vi "Measurement Logic.vi"() -> ()   [LabVIEW 2024, in "NIScopeTimeDomain.lvlib"]
uses:
  NIScopeTimeDomain.lvlib
  Measurement Configuration.ctl
  <vilib>/MeasurementLink/MeasurementLink Measurement Server/Measure Call Context/Measure Call Context.lvclass
  Measurement Results.ctl
  <instrlib>/niScope/Controls/niScope scalar measurement.ctl
  <vilib>/MeasurementLink/MeasurementLink Measurement Server/Measure Call Context/Reserve Sessions - 1Pin.vi
  <vilib>/MeasurementLink/MeasurementLink niScope/Initialize Sessions - 1Sess.vi
  <vilib>/MeasurementLink/MeasurementLink niScope/Get Connections - 1Pin 1Conn.vi
  <instrlib>/niScope/Configure/Trigger/niScope Configure Trigger Edge.vi
  <instrlib>/niScope/Acquire/Fetch/niScope Fetch WDT.vi
  <instrlib>/niScope/Measurements/niScope Fetch Measurement Stats.vi
  <vilib>/MeasurementLink/MeasurementLink niScope/MeasurementLink niScope.lvlib
  <vilib>/MeasurementLink/MeasurementLink Session Management V1/Session Reservation/Session Reservation.lvclass
panel:
  out "measurement results":T1
  out "measure call context out":refnum<class "Measure Call Context.lvclass">
  in  "measure call context in":refnum<class "Measure Call Context.lvclass">
  in  "measurement configuration":T2={"Pin Name"="", "Vertical Range (V)"=10.0, "Vertical Offset (V)"=0.0, "Vertical Coupling"=1, "Minimum Sample Rate (S/s)"=10000000.0, "Minimum Record Length (S)"=40000.0, "Trigger Level (V)"=0.5, "Trigger Coupling"=0, "Trigger Slope"=1} {"Trigger Slope" items=["AC"=0, "DC"=1, "HF Reject"=3, "LF Reject"=4, "AC Plus HF Reject"=1001]; "Trigger Coupling" items=["Positive", "Negative"]; "Vertical Coupling" items=["AC", "DC", "Ground"]; "Vertical Offset (V)" format="%.2p"}
  out "error out":errorcluster
  in  "error in":errorcluster
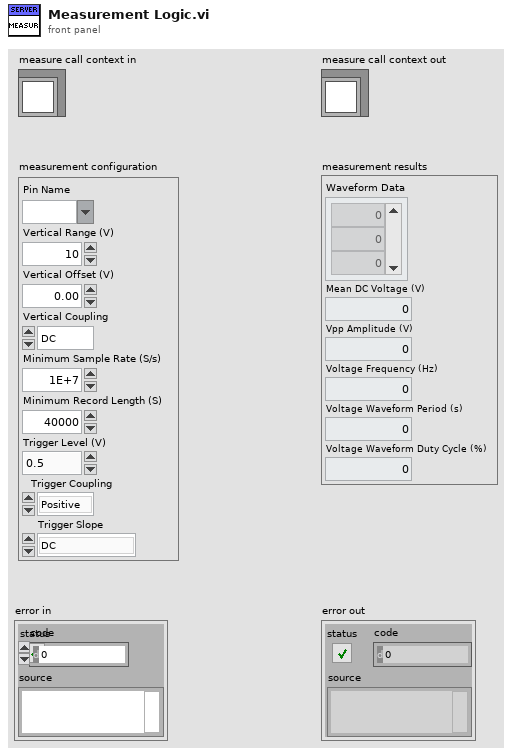
[diagram p1: front panel]
types:
  T1 = typedef "NIScopeTimeDomain.lvlib/Measurement Results.ctl" = cluster{"Waveform Data":dbl[], "Mean DC Voltage (V)":dbl, "Vpp Amplitude (V)":dbl, "Voltage Frequency (Hz)":dbl, "Voltage Waveform Period (s)":dbl, "Voltage Waveform Duty Cycle (%)":dbl}
  T2 = typedef "NIScopeTimeDomain.lvlib/Measurement Configuration.ctl" = cluster{"Pin Name":string, "Vertical Range (V)":dbl, "Vertical Offset (V)":dbl, "Vertical Coupling":i32, "Minimum Sample Rate (S/s)":dbl, "Minimum Record Length (S)":dbl, "Trigger Level (V)":dbl, "Trigger Coupling":u32, "Trigger Slope":i32}
  T3 = typedef "niScope scalar measurement.ctl" = i32
  T4 = typedef "MeasurementLink niScope.lvlib/Connection with Session.ctl" = cluster{"connection":T5, "session":refnum<k15>}
  T5 = typedef "MeasurementLink Session Management V1.lvlib/Session Reservation.lvclass/Connection.ctl" = cluster{"pin or relay name":string, "site":i32, "instrument type id":string, "channel":string}
  T6 = cluster{"result":dbl, "mean":dbl, "stdev":dbl, "min":dbl, "max":dbl, "num in stats":i32}
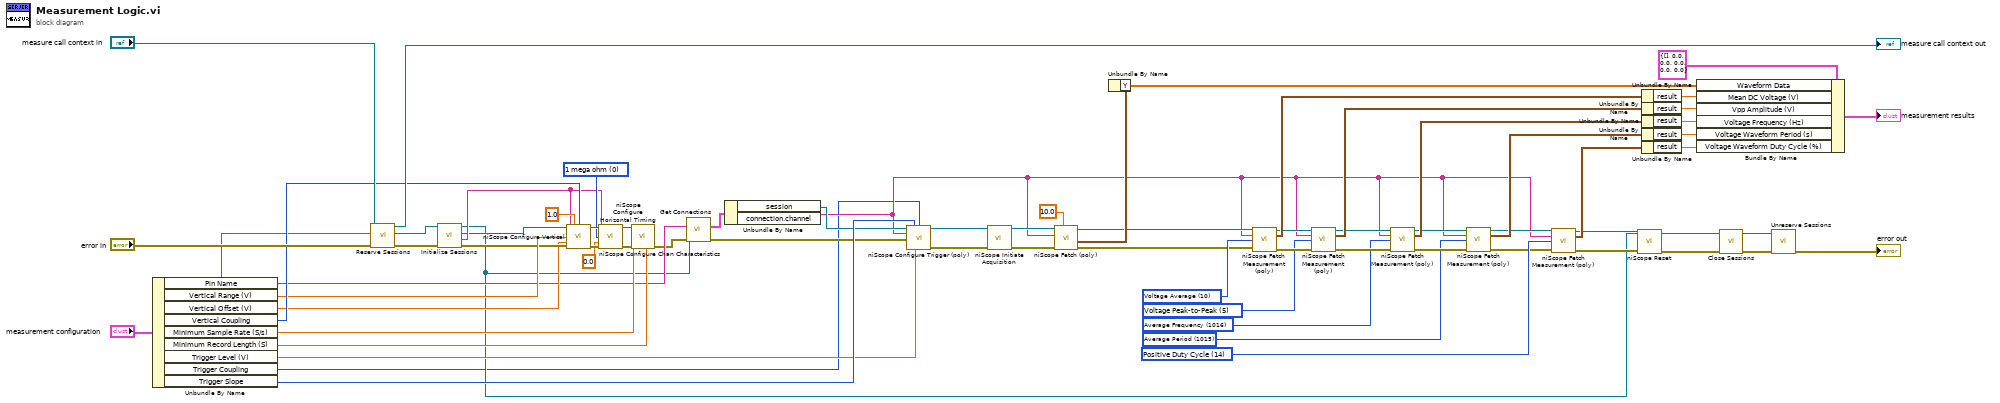
[diagram p0: block diagram]
diagram:
  w8 = T3 1015 items=["None"=4000, "Frequency"=2, "Average Frequency"=1016, "FFT Frequency"=1008, "Period"=3, "Average Period"=1015, "Rise Time"=0, "Fall Time"=1, "Rising Slew Rate"=1010, "Falling Slew Rate"=1011, "Overshoot"=18, "Preshoot"=19, "Voltage RMS"=4, "Voltage Cycle RMS"=16, "AC Estimate"=1012, "FFT Amplitude"=1009, "Voltage Average"=10, "Voltage Cycle Average"=17, "DC Estimate"=1013, "Voltage Max"=6, "Voltage Min"=7, "Voltage Peak-to-Peak"=5, "Voltage High"=8, "Voltage Low"=9, "Voltage Amplitude"=15, "Voltage Top"=1007, "Voltage Base"=1006, "Voltage Base-to-Top"=1017, "Negative Width"=11, "Positive Width"=12, "Negative Duty Cycle"=13, "Positive Duty Cycle"=14, "Integral"=1005, "Area"=1003, "Cycle Area"=1004, "Time Delay"=1014, "Phase Delay"=1018, "Low Ref Volts"=1000, "Mid Ref Volts"=1001, "High Ref Volts"=1002, "Volt. Hist. Mean"=2000, "Volt. Hist. Stdev"=2001, "Volt. Hist. Median"=2003, "Volt. Hist. Mode"=2010, "Volt. Hist. Max"=2005, "Volt. Hist. Min"=2006, "Volt. Hist. Peak-to-Peak"=2002, "Volt. Hist. Mean + Stdev"=2007, "Volt. Hist. Mean + 2 Stdev"=2008, "Volt. Hist. Mean + 3 Stdev"=2009, "Volt. Hist. Hits"=2004, "Volt. Hist. New Hits"=2011, "Time Hist. Mean"=3000, "Time Hist. Stdev"=3001, "Time Hist. Median"=3003, "Time Hist. Mode"=3010, "Time Hist. Max"=3005, "Time Hist. Min"=3006, "Time Hist. Peak-to-Peak"=3002, "Time Hist. Mean + Stdev"=3007, "Time Hist. Mean + 2 Stdev"=3008, "Time Hist. Mean + 3 Stdev"=3009, "Time Hist. Hits"=3004, "Time Hist. New Hits"=3011] ("scalar measurement")
  w19 = T3 14 items=["None"=4000, "Frequency"=2, "Average Frequency"=1016, "FFT Frequency"=1008, "Period"=3, "Average Period"=1015, "Rise Time"=0, "Fall Time"=1, "Rising Slew Rate"=1010, "Falling Slew Rate"=1011, "Overshoot"=18, "Preshoot"=19, "Voltage RMS"=4, "Voltage Cycle RMS"=16, "AC Estimate"=1012, "FFT Amplitude"=1009, "Voltage Average"=10, "Voltage Cycle Average"=17, "DC Estimate"=1013, "Voltage Max"=6, "Voltage Min"=7, "Voltage Peak-to-Peak"=5, "Voltage High"=8, "Voltage Low"=9, "Voltage Amplitude"=15, "Voltage Top"=1007, "Voltage Base"=1006, "Voltage Base-to-Top"=1017, "Negative Width"=11, "Positive Width"=12, "Negative Duty Cycle"=13, "Positive Duty Cycle"=14, "Integral"=1005, "Area"=1003, "Cycle Area"=1004, "Time Delay"=1014, "Phase Delay"=1018, "Low Ref Volts"=1000, "Mid Ref Volts"=1001, "High Ref Volts"=1002, "Volt. Hist. Mean"=2000, "Volt. Hist. Stdev"=2001, "Volt. Hist. Median"=2003, "Volt. Hist. Mode"=2010, "Volt. Hist. Max"=2005, "Volt. Hist. Min"=2006, "Volt. Hist. Peak-to-Peak"=2002, "Volt. Hist. Mean + Stdev"=2007, "Volt. Hist. Mean + 2 Stdev"=2008, "Volt. Hist. Mean + 3 Stdev"=2009, "Volt. Hist. Hits"=2004, "Volt. Hist. New Hits"=2011, "Time Hist. Mean"=3000, "Time Hist. Stdev"=3001, "Time Hist. Median"=3003, "Time Hist. Mode"=3010, "Time Hist. Max"=3005, "Time Hist. Min"=3006, "Time Hist. Peak-to-Peak"=3002, "Time Hist. Mean + Stdev"=3007, "Time Hist. Mean + 2 Stdev"=3008, "Time Hist. Mean + 3 Stdev"=3009, "Time Hist. Hits"=3004, "Time Hist. New Hits"=3011] ("scalar measurement")
  w20 = T3 1016 items=["None"=4000, "Frequency"=2, "Average Frequency"=1016, "FFT Frequency"=1008, "Period"=3, "Average Period"=1015, "Rise Time"=0, "Fall Time"=1, "Rising Slew Rate"=1010, "Falling Slew Rate"=1011, "Overshoot"=18, "Preshoot"=19, "Voltage RMS"=4, "Voltage Cycle RMS"=16, "AC Estimate"=1012, "FFT Amplitude"=1009, "Voltage Average"=10, "Voltage Cycle Average"=17, "DC Estimate"=1013, "Voltage Max"=6, "Voltage Min"=7, "Voltage Peak-to-Peak"=5, "Voltage High"=8, "Voltage Low"=9, "Voltage Amplitude"=15, "Voltage Top"=1007, "Voltage Base"=1006, "Voltage Base-to-Top"=1017, "Negative Width"=11, "Positive Width"=12, "Negative Duty Cycle"=13, "Positive Duty Cycle"=14, "Integral"=1005, "Area"=1003, "Cycle Area"=1004, "Time Delay"=1014, "Phase Delay"=1018, "Low Ref Volts"=1000, "Mid Ref Volts"=1001, "High Ref Volts"=1002, "Volt. Hist. Mean"=2000, "Volt. Hist. Stdev"=2001, "Volt. Hist. Median"=2003, "Volt. Hist. Mode"=2010, "Volt. Hist. Max"=2005, "Volt. Hist. Min"=2006, "Volt. Hist. Peak-to-Peak"=2002, "Volt. Hist. Mean + Stdev"=2007, "Volt. Hist. Mean + 2 Stdev"=2008, "Volt. Hist. Mean + 3 Stdev"=2009, "Volt. Hist. Hits"=2004, "Volt. Hist. New Hits"=2011, "Time Hist. Mean"=3000, "Time Hist. Stdev"=3001, "Time Hist. Median"=3003, "Time Hist. Mode"=3010, "Time Hist. Max"=3005, "Time Hist. Min"=3006, "Time Hist. Peak-to-Peak"=3002, "Time Hist. Mean + Stdev"=3007, "Time Hist. Mean + 2 Stdev"=3008, "Time Hist. Mean + 3 Stdev"=3009, "Time Hist. Hits"=3004, "Time Hist. New Hits"=3011] ("scalar measurement")
  w23 = T3 5 items=["None"=4000, "Frequency"=2, "Average Frequency"=1016, "FFT Frequency"=1008, "Period"=3, "Average Period"=1015, "Rise Time"=0, "Fall Time"=1, "Rising Slew Rate"=1010, "Falling Slew Rate"=1011, "Overshoot"=18, "Preshoot"=19, "Voltage RMS"=4, "Voltage Cycle RMS"=16, "AC Estimate"=1012, "FFT Amplitude"=1009, "Voltage Average"=10, "Voltage Cycle Average"=17, "DC Estimate"=1013, "Voltage Max"=6, "Voltage Min"=7, "Voltage Peak-to-Peak"=5, "Voltage High"=8, "Voltage Low"=9, "Voltage Amplitude"=15, "Voltage Top"=1007, "Voltage Base"=1006, "Voltage Base-to-Top"=1017, "Negative Width"=11, "Positive Width"=12, "Negative Duty Cycle"=13, "Positive Duty Cycle"=14, "Integral"=1005, "Area"=1003, "Cycle Area"=1004, "Time Delay"=1014, "Phase Delay"=1018, "Low Ref Volts"=1000, "Mid Ref Volts"=1001, "High Ref Volts"=1002, "Volt. Hist. Mean"=2000, "Volt. Hist. Stdev"=2001, "Volt. Hist. Median"=2003, "Volt. Hist. Mode"=2010, "Volt. Hist. Max"=2005, "Volt. Hist. Min"=2006, "Volt. Hist. Peak-to-Peak"=2002, "Volt. Hist. Mean + Stdev"=2007, "Volt. Hist. Mean + 2 Stdev"=2008, "Volt. Hist. Mean + 3 Stdev"=2009, "Volt. Hist. Hits"=2004, "Volt. Hist. New Hits"=2011, "Time Hist. Mean"=3000, "Time Hist. Stdev"=3001, "Time Hist. Median"=3003, "Time Hist. Mode"=3010, "Time Hist. Max"=3005, "Time Hist. Min"=3006, "Time Hist. Peak-to-Peak"=3002, "Time Hist. Mean + Stdev"=3007, "Time Hist. Mean + 2 Stdev"=3008, "Time Hist. Mean + 3 Stdev"=3009, "Time Hist. Hits"=3004, "Time Hist. New Hits"=3011] ("scalar measurement")
  w31 = T3 10 items=["None"=4000, "Frequency"=2, "Average Frequency"=1016, "FFT Frequency"=1008, "Period"=3, "Average Period"=1015, "Rise Time"=0, "Fall Time"=1, "Rising Slew Rate"=1010, "Falling Slew Rate"=1011, "Overshoot"=18, "Preshoot"=19, "Voltage RMS"=4, "Voltage Cycle RMS"=16, "AC Estimate"=1012, "FFT Amplitude"=1009, "Voltage Average"=10, "Voltage Cycle Average"=17, "DC Estimate"=1013, "Voltage Max"=6, "Voltage Min"=7, "Voltage Peak-to-Peak"=5, "Voltage High"=8, "Voltage Low"=9, "Voltage Amplitude"=15, "Voltage Top"=1007, "Voltage Base"=1006, "Voltage Base-to-Top"=1017, "Negative Width"=11, "Positive Width"=12, "Negative Duty Cycle"=13, "Positive Duty Cycle"=14, "Integral"=1005, "Area"=1003, "Cycle Area"=1004, "Time Delay"=1014, "Phase Delay"=1018, "Low Ref Volts"=1000, "Mid Ref Volts"=1001, "High Ref Volts"=1002, "Volt. Hist. Mean"=2000, "Volt. Hist. Stdev"=2001, "Volt. Hist. Median"=2003, "Volt. Hist. Mode"=2010, "Volt. Hist. Max"=2005, "Volt. Hist. Min"=2006, "Volt. Hist. Peak-to-Peak"=2002, "Volt. Hist. Mean + Stdev"=2007, "Volt. Hist. Mean + 2 Stdev"=2008, "Volt. Hist. Mean + 3 Stdev"=2009, "Volt. Hist. Hits"=2004, "Volt. Hist. New Hits"=2011, "Time Hist. Mean"=3000, "Time Hist. Stdev"=3001, "Time Hist. Median"=3003, "Time Hist. Mode"=3010, "Time Hist. Max"=3005, "Time Hist. Min"=3006, "Time Hist. Peak-to-Peak"=3002, "Time Hist. Mean + Stdev"=3007, "Time Hist. Mean + 2 Stdev"=3008, "Time Hist. Mean + 3 Stdev"=3009, "Time Hist. Hits"=3004, "Time Hist. New Hits"=3011] ("scalar measurement")
  w55 = u32 0 items=["1 mega ohm"=0, "50 ohms"=2] ("input impedance")
  n1 = Unbundle By Name("measurement configuration") -> ("Pin Name"=w36:string, "Vertical Range (V)"=w61:dbl, "Vertical Offset (V)"=w59:dbl, "Vertical Coupling"=w65:i32, "Minimum Sample Rate (S/s)"=w52:dbl, "Minimum Record Length (S)"=w50:dbl, "Trigger Level (V)"=w48:dbl, "Trigger Coupling"=w1:u32, "Trigger Slope"=w49:i32)
  n2 = call-poly <vilib>:"Reserve Sessions.vi"("error in"="error in", "pin or relay name"=w36, "measurement context in"="measure call context in") -> ("error out"=w67:errorcluster, "session reservation out"=w68:refnum<class "Session Reservation.lvclass">, "measurement context out"=→"measure call context out":refnum<class "Measure Call Context.lvclass">)  [unwired: 6 in]
  n3 = call-poly <vilib>:"Initialize Sessions.vi"("error in"=w67, "session reservation in"=w68) -> ("error out"=w60:errorcluster, "channel list"=w53:string, "session"=w46:refnum<k15>, "session reservation out"=w2:refnum<class "Session Reservation.lvclass">)  [unwired: 6 in]
  n4 = call <instrlib>:"niScope Configure Vertical.vi"("instrument handle"=w46, "probe attenuation"=1.0, "vertical coupling"=w65, "channels"=w53, "vertical range"=w61, "vertical offset"=w59, "error in"=w60) -> ("instrument handle out"=w57:refnum<k15>, "error out"=w56:errorcluster)  [unwired: 7 in]
  n5 = call <instrlib>:"niScope Configure Chan Characteristics.vi"("instrument handle"=w57, "channels"=w53, "input impedance"=w55, "maximum input frequency"=0.0, "error in"=w56) -> ("instrument handle out"=w41:refnum<k15>, "error out"=w51:errorcluster)  [unwired: 9 in]
  n6 = call <instrlib>:"niScope Configure Horizontal Timing.vi"("instrument handle"=w41, "min sample rate"=w52, "error in"=w51, "min record length"=w50) -> ("error out"=w35:errorcluster)  [unwired: 10 in, 1 out]
  n7 = call-poly <vilib>:"Get Connections.vi"("error in"=w35, "pin or relay name"=w36, "session reservation in"=w2) -> ("error out"=w34:errorcluster, "connection"=w33:T4)  [unwired: 6 in, 1 out]
  n8 = Unbundle By Name(w33) -> ("session"=w32:refnum<k15>, "connection.channel"=w3:string)
  n9 = call-poly <instrlib>:"niScope Configure Trigger (poly).vi"("instrument handle"=w32, "trigger slope"=w49, "trigger coupling"=w1, "trigger source"=w3, "trigger level"=w48, "error in"=w34) -> ("instrument handle out"=w45:refnum<k15>, "error out"=w47:errorcluster)  [unwired: 8 in]
  n10 = call <instrlib>:"niScope Initiate Acquisition.vi"("instrument handle"=w45, "error in"=w47) -> ("instrument handle out"=w44:refnum<k15>, "error out"=w43:errorcluster)  [unwired: 12 in]
  n11 = call-poly <instrlib>:"niScope Fetch (poly).vi"("timeout"=10.0, "error in"=w43, "channels"=w3, "instrument handle"=w44) -> ("error out"=w28:errorcluster, "wfm"=w40:waveform(dbl), "instrument handle out"=w7:refnum<k15>)  [unwired: 4 in, 1 out]
  n12 = Unbundle By Name(w40) -> ("Y"=w39:dbl[])
  n13 = call-poly <instrlib>:"niScope Fetch Measurement (poly).vi"("instrument handle"=w7, "channels"=w3, "scalar measurement"=w31, "error in"=w28) -> ("instrument handle out"=w27:refnum<k15>, "stats"=w30:T6, "error out"=w24:errorcluster)  [unwired: 9 in]
  n14 = call-poly <instrlib>:"niScope Fetch Measurement (poly).vi"("instrument handle"=w27, "channels"=w3, "scalar measurement"=w23, "error in"=w24) -> ("instrument handle out"=w22:refnum<k15>, "stats"=w26:T6, "error out"=w21:errorcluster)  [unwired: 9 in]
  n15 = call-poly <instrlib>:"niScope Fetch Measurement (poly).vi"("instrument handle"=w22, "channels"=w3, "scalar measurement"=w20, "error in"=w21) -> ("instrument handle out"=w9:refnum<k15>, "stats"=w18:T6, "error out"=w13:errorcluster)  [unwired: 9 in]
  n16 = call-poly <instrlib>:"niScope Fetch Measurement (poly).vi"("instrument handle"=w9, "channels"=w3, "scalar measurement"=w8, "error in"=w13) -> ("instrument handle out"=w10:refnum<k15>, "stats"=w11:T6, "error out"=w14:errorcluster)  [unwired: 9 in]
  n17 = call-poly <instrlib>:"niScope Fetch Measurement (poly).vi"("instrument handle"=w10, "channels"=w3, "scalar measurement"=w19, "error in"=w14) -> ("instrument handle out"=w5:refnum<k15>, "stats"=w15:T6, "error out"=w4:errorcluster)  [unwired: 9 in]
  n18 = call <instrlib>:"niScope Reset.vi"("instrument handle"=w5, "error in"=w4) -> ("error out"=w6:errorcluster)  [unwired: 12 in, 1 out]
  n19 = Unbundle By Name(w30) -> ("result"=w29:dbl)
  n20 = Unbundle By Name(w26) -> ("result"=w25:dbl)
  n21 = Unbundle By Name(w18) -> ("result"=w17:dbl)
  n22 = Unbundle By Name(w11) -> ("result"=w12:dbl)
  n23 = Unbundle By Name(w15) -> ("result"=w16:dbl)
  n24 = Bundle By Name(cluster=T1 {"Waveform Data"=[], "Mean DC Voltage (V)"=0.0, "Vpp Amplitude (V)"=0.0, "Voltage Frequency (Hz)"=0.0, "Voltage Waveform Period (s)"=0.0, "Voltage Waveform Duty Cycle (%)"=0.0} ("measurement results"), "Waveform Data"=w39, "Mean DC Voltage (V)"=w29, "Vpp Amplitude (V)"=w25, "Voltage Frequency (Hz)"=w17, "Voltage Waveform Period (s)"=w12, "Voltage Waveform Duty Cycle (%)"=w16) -> (→"measurement results":T1)
  n25 = call <vilib>:"Close Sessions.vi"("error in"=w6, "session reservation in"=w2) -> ("error out"=w62:errorcluster, "session reservation out"=w64:refnum<class "Session Reservation.lvclass">)  [unwired: 8 in]
  n26 = call <vilib>:"Unreserve Sessions.vi"("error in"=w62, "session reservation in"=w64) -> ("error out"=→"error out":errorcluster)  [unwired: 9 in]
